vi "Set Sampling Rate.vi"(8 "error in (no error)":errorcluster, 11 "LINX-ADS1256 in":refnum<class "LINX-ADS1256.lvclass">) -> (0 "error out":errorcluster, 3 "LINX-ADS1256 out":refnum<class "LINX-ADS1256.lvclass">)   [LabVIEW 2020, in "LINX-ADS1256.lvclass"]
uses:
  LINX-ADS1256.lvclass
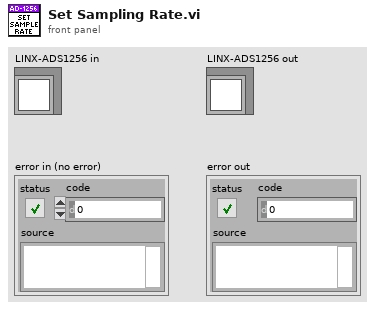
[diagram p1: front panel]
types:
  T1 = typedef "LINX-ADS1256.lvclass/Sample Rate.ctl" = enum16{"2.5Hz", "5Hz", "10Hz", "15Hz", "25Hz", "30Hz", "50Hz", "60Hz", "100Hz", "500Hz", "1000Hz", "2000Hz", "3750Hz", "7500Hz", "15000Hz", "30000Hz"}
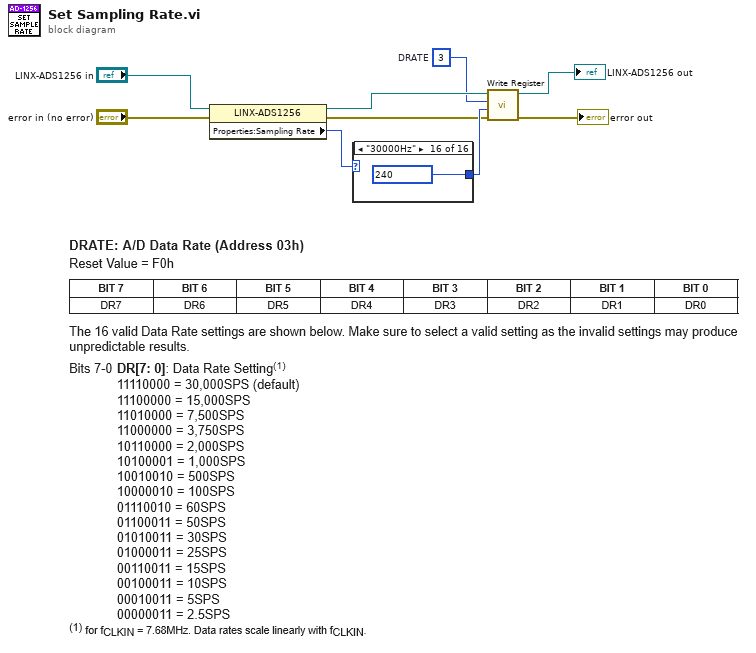
[diagram p0: block diagram]
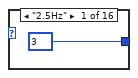
[diagram p2: hidden frame]
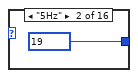
[diagram p3: hidden frame]
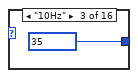
[diagram p4: hidden frame]
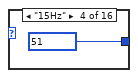
[diagram p5: hidden frame]
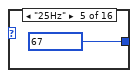
[diagram p6: hidden frame]
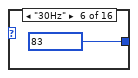
[diagram p7: hidden frame]
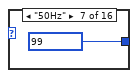
[diagram p8: hidden frame]
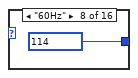
[diagram p9: hidden frame]
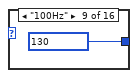
[diagram p10: hidden frame]
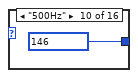
[diagram p11: hidden frame]
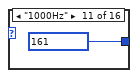
[diagram p12: hidden frame]
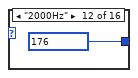
[diagram p13: hidden frame]
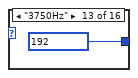
[diagram p14: hidden frame]
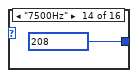
[diagram p15: hidden frame]
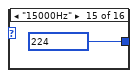
[diagram p16: hidden frame]
diagram:
  w2 = u8 3  # DRATE
  n1 = property class="LINX-ADS1256"(reference="LINX-ADS1256 in", error in="error in (no error)") -> (reference out=w4:refnum<class "LINX-ADS1256.lvclass">, error out=w5:errorcluster, "Properties:Sampling Rate"=w8:T1)
  n2 = case shown="\"30000Hz\"" w8 {
    tunnel: [u8 3 u8 19 u8 35 u8 51 u8 67 u8 83 u8 99 u8 114 u8 130 u8 146 u8 161 u8 176 u8 192 u8 208 u8 224 u8 240] -> w9
    frame "2.5Hz" {
    }
    frame "5Hz" {
    }
    frame "10Hz" {
    }
    frame "15Hz" {
    }
    frame "25Hz" {
    }
    frame "30Hz" {
    }
    frame "50Hz" {
    }
    frame "60Hz" {
    }
    frame "100Hz" {
    }
    frame "500Hz" {
    }
    frame "1000Hz" {
    }
    frame "2000Hz" {
    }
    frame "3750Hz" {
    }
    frame "7500Hz" {
    }
    frame "15000Hz" {
    }
    frame "30000Hz" {
    }
  }
  n3 = call "Write Register.vi"("error in (no error)"=w5, "Data"=w9, "Register Address"=w2, "LINX-ADS1256 in"=w4) -> ("error out"=→"error out":errorcluster, "LINX-ADS1256 out"=→"LINX-ADS1256 out":refnum<class "LINX-ADS1256.lvclass">)  [unwired: 6 in]
